vi "Deinit.vi"(0 "SystemEvents in":refnum<class "SystemEvents.lvclass">, 5 "error in (no error)":errorcluster) -> (14 "SystemEvents out":refnum<class "SystemEvents.lvclass">, 19 "error out":errorcluster)   [LabVIEW 2017, in "SystemEvents.lvclass"]
doc: "Destroys the user events in the 'Events' object attribute."
uses:
  SystemEvents.lvclass
  SystemEvents.lvclass/SystemEvents.ctl
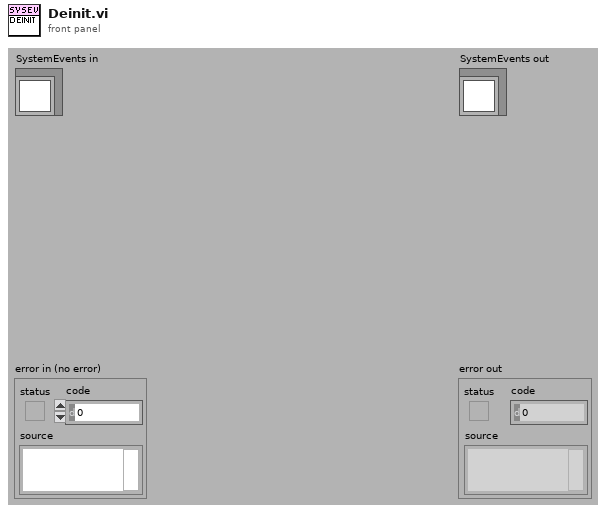
[diagram p1: front panel]
types:
  T1 = typedef "SystemEventsType.ctl" = cluster{"TrigOn":refnum<user-event>, "TrigOff":refnum<user-event>, "Result":refnum<user-event>, "Enable":refnum<user-event>, "Stop":refnum<user-event>, "AnalysisCompleted":refnum<user-event>, "Info":refnum<user-event>}
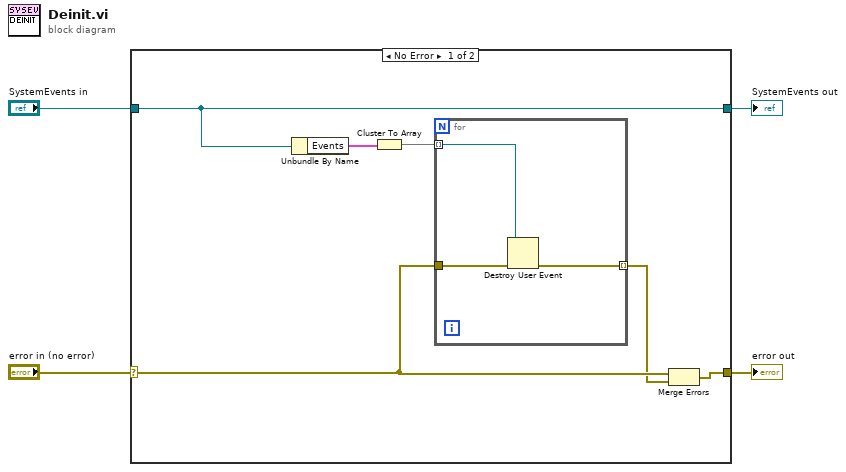
[diagram p0: block diagram]
diagram:
  n1 = case shown="No Error" "error in (no error)" {
    selector: "error in (no error)" -> [w7 w15]
    tunnel: [w6 w15] -> w3
    tunnel: [w10 w14] -> w1
    tunnel: "SystemEvents in" -> [w10 w14]
    frame No Error {
      n2 = Unbundle By Name(w10) -> ("Events"=w9:T1)
      n3 = Cluster To Array(cluster=w9) -> (array=w8:refnum<user-event>[])
      n4 = for {
        tunnel: w8 -> [w13] mode=indexing
        tunnel: w7 -> [w12]
        tunnel: [w11] -> w5 mode=indexing
        n5 = Destroy User Event(user event=w13, error in=w12) -> (error out=w11:errorcluster)
      }
      n6 = Merge Errors(w7, w5) -> (w6:errorcluster)
    }
    frame Error {
    }
  }
  "error out" <- w3
  "SystemEvents out" <- w1
